vi "ST Cmd.vi"(5 "error in (no error)":errorcluster, 6 "Time Out":i32=10000, 7 "Command String":string, 8 "VISA resource name":refnum<visa-resource-name>="COM1") -> (0 "error out":errorcluster, 1 "String Received":string, 2 "Ready and OK":bool, 3 "VISA resource name out":refnum<visa-resource-name>, 4 "Result Code":i32)   [LabVIEW 2009]
doc: "This VI accepts a command, adds carriage return and line feed, and sends to ST Robotic via the Com line.\nIt reads the return string, with a True on the Ready and OK and a result code for other results. The result out has the following meaning:\n 0 >>> Operation not complete\n 1 >>> Operation Complete with an Error\n 2 >>> Operation Complete without Error\n-1 >>> Operation caused a Communication Error"
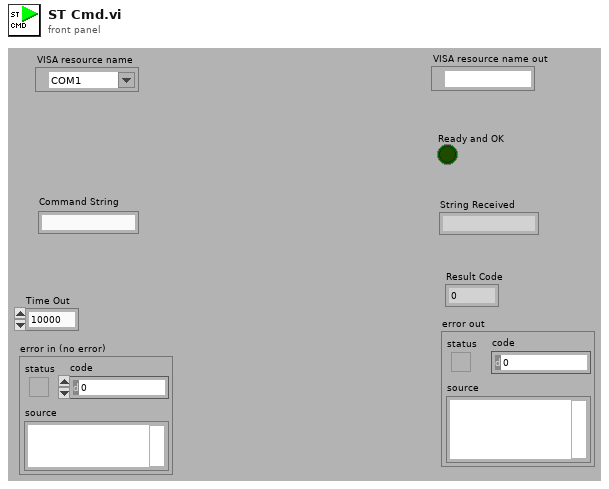
[diagram p1: front panel]
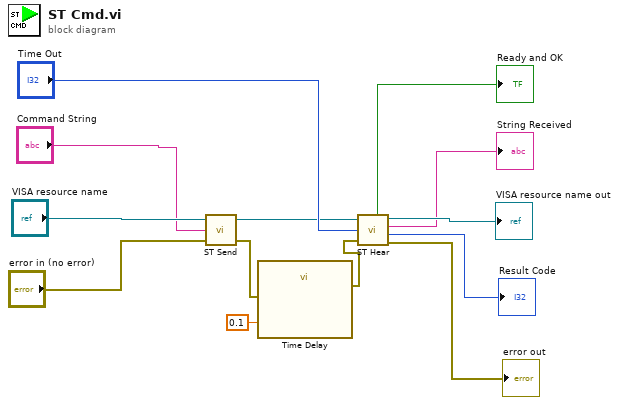
[diagram p0: block diagram]
diagram:
  n1 = call "ST Send.vi"("error in (no error)"="error in (no error)", "String"="Command String", "VISA resource name"="VISA resource name") -> ("error out"=w3:errorcluster, "VISA resource name out"=w12:refnum<visa-resource-name>)  [unwired: 1 out]
  n2 = call "Time Delay"("error in (no error)"=w3, "Delay Time (s)"=0.1) -> ("error out"=w2:errorcluster)  [unwired: 9 in]
  n3 = call "ST Hear.vi"("VISA resource name"=w12, "Time Out"="Time Out", "error in (no error)"=w2) -> ("VISA resource name out"=→"VISA resource name out":refnum<visa-resource-name>, "String Received"=→"String Received":string, "Result Code"=→"Result Code":i32, "error out"=→"error out":errorcluster, "Ready and OK"=→"Ready and OK":bool)
